vi "Funnel_Notifier_Begin.vi"   [LabVIEW 2020]
uses:
  Globals/Funnel_global.vi
  Control_states_funnle.ctl
  Cluster_funnel.ctl
types:
  T1 = typedef "Cluster_funnel.ctl" = cluster{"Control States":T2, "On?":bool}
  T2 = typedef "Control_states_funnle.ctl" = enum16{"no_op", "ball_op"}
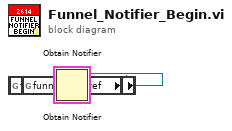
[diagram p0: block diagram]
diagram:
  w3 = T1 {"Control States"=enum."no_op", "On?"=FALSE}
  n1 = global read "Funnel_global.vi" "funnel_execute_ref"() -> (w1:string)
  n2 = global read "Funnel_global.vi" "funnel_set_ref"() -> (w2:string)
  n3 = Obtain Notifier(name (unnamed)=w1, notification data type=w3) -> (notifier out=w4:refnum<notifier>)  [unwired: 2 in, 2 out]
  n4 = global write "Funnel_global.vi" "Funnel_execute_ref"(w4) -> ()
  n5 = Obtain Notifier(name (unnamed)=w2, notification data type=w3) -> (notifier out=w5:refnum<notifier>)  [unwired: 2 in, 2 out]
  n6 = global write "Funnel_global.vi" "Funnel_set_ref"(w5) -> ()
